vi "Define 2D Helmholtz PDE (Numeric).vi"(0 "PDE in":refnum<class "NI_PDE.lvclass">, 5 "F(x, y)":dbl[][](array[numeric]), 7 "k":dbl=1.0, 9 "a":dbl, 11 "error in (no error)":errorcluster) -> (4 "PDE out":refnum<class "NI_PDE.lvclass">, 15 "error out":errorcluster)   [LabVIEW 2017, in "NI_PDE.lvlib"]
doc: "Defines the right side of a partial differential equation and its coefficients. You must manually select the polymorphic instance to use."
uses:
  <vilib>/gmath/NI_PDE.lvlib
  <vilib>/gmath/pde.llb/PDEClass/NI_PDE.lvclass
  <vilib>/gmath/pde.llb/PDEClass/PDE_Helmholtz_2D/NI_PDE_Helmholtz_2D.lvclass
  e:/builds/penguin/labview/branches/2017/dev/dist/vi.lib/gmath/pde.llb/PDEClass/NI_PDE.lvclass
  <vilib>/gmath/pde.llb/RHSClass/RHS_2D_Numeric/NI_RHS_2D_Numeric.lvclass
  e:/builds/penguin/labview/branches/2017/dev/dist/vi.lib/gmath/pde.llb/RHSClass/NI_RHS.lvclass
  <vilib>/gmath/pde.llb/PDEClass/PDE_2ndOrder_ConstPara/Para Data.ctl
  <vilib>/gmath/pde.llb/PDEClass/PDE_2ndOrder_ConstPara/NI_PDE_2ndOrder_ConstPara.lvclass
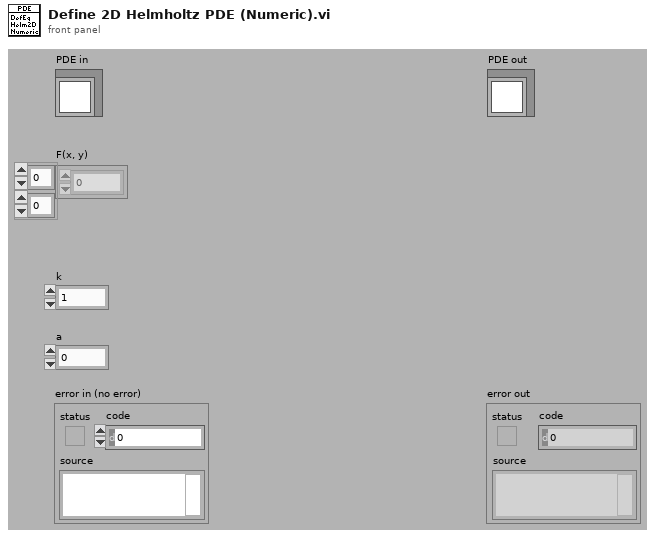
[diagram p1: front panel]
types:
  T1 = typedef "NI_PDE.lvlib/NI_PDE_2ndOrder_ConstPara.lvclass/Para Data.ctl" = cluster{"k":dbl, "a":dbl}
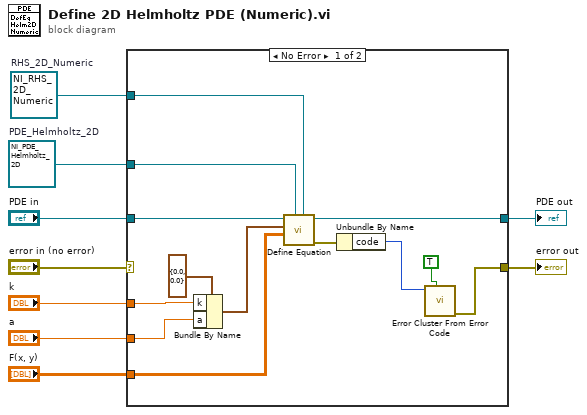
[diagram p0: block diagram]
diagram:
  w1 = refnum<class "NI_RHS_2D_Numeric.lvclass"> refnum  # RHS_2D_Numeric
  w2 = refnum<class "NI_PDE_Helmholtz_2D.lvclass"> refnum  # PDE_Helmholtz_2D
  n1 = case shown="No Error" "error in (no error)" {
    selector: "error in (no error)" -> [_ w23]
    tunnel: "PDE in" -> [w14 w24]
    tunnel: [w13 w24] -> w8
    tunnel: [w21 w23] -> w7
    tunnel: "F(x, y)" -> [w10 _]
    tunnel: "a" -> [w17 _]
    tunnel: "k" -> [w18 _]
    tunnel: w2 -> [w16 _]
    tunnel: w1 -> [w15 _]
    frame No Error {
      n2 = Bundle By Name(cluster=T1 {"k"=0.0, "a"=0.0} ("const para"), "k"=w18, "a"=w17) -> (w12:T1)
      n3 = call <vilib>:"Define Equation.vi"("target RHS"=w15, "target PDE"=w16, "RHS"=w10, "parameter"=w12, "PDE in"=w14) -> ("error out"=w11:errorcluster, "PDE out"=w13:refnum<class "NI_PDE.lvclass">)  [unwired: 1 in, 4 out]
      n4 = Unbundle By Name(w11) -> ("code"=w22:i32)
      n5 = call <vilib>:"Error Cluster From Error Code.vi"("show call chain? (False)"=TRUE, "error code (0)"=w22) -> ("error out"=w21:errorcluster)  [unwired: 1 in, 6 out]
    }
    frame Error {
    }
  }
  "PDE out" <- w8
  "error out" <- w7
